vi "load setup.vi"(8 "错误输入（无错误）":errorcluster, 10 "path":path, 11 "VISA GPIB Resource":refnum<visa-resource-name>="GPIB0::2::INSTR" caption="VISA GPIB资源") -> (0 "错误输出":errorcluster, 3 "VISA资源名称输出":refnum<visa-resource-name>)   [LabVIEW 2017]
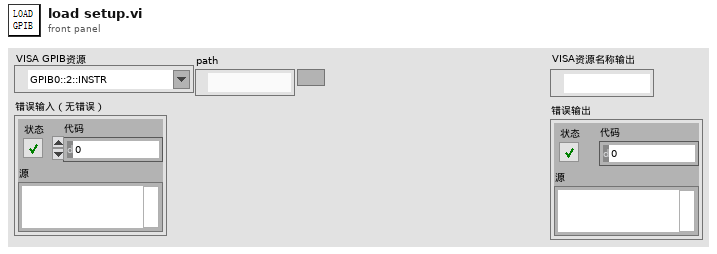
[diagram p1: front panel]
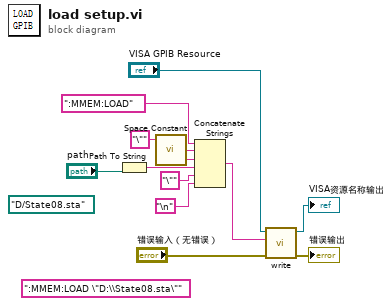
[diagram p0: block diagram]
diagram:
  (unwired) path "D:/State08.sta" ("路径")
  (unwired) ":MMEM:LOAD \"D:\\State08.sta\""
  n1 = Path To String(path="path") -> (string=w7:string)
  n2 = call <vilib>:"Space Constant.vi"() -> ("String"=w3:string)
  n3 = Concatenate Strings(":MMEM:LOAD" ("字符串"), w3, "\"" ("字符串"), w7, "\"" ("字符串"), "\n") -> (w1:string)
  n4 = call "write.vi"("错误输入（无错误）"="错误输入（无错误）", "Write Buffer"=w1, "VISA GPIB Resource"="VISA GPIB Resource") -> ("错误输出"=→"错误输出":errorcluster, "VISA资源名称输出"=→"VISA资源名称输出":refnum<visa-resource-name>)  [unwired: 7 in]
